vi "mrq_getdi.vi"(3 "错误输入（无错误）":errorcluster, 6 "VISA资源名称":refnum<visa-resource-name>) -> (0 "错误输出":errorcluster, 1 "数字":i32, 2 "VISA资源名称输出":refnum<visa-resource-name>)   [LabVIEW 2017]
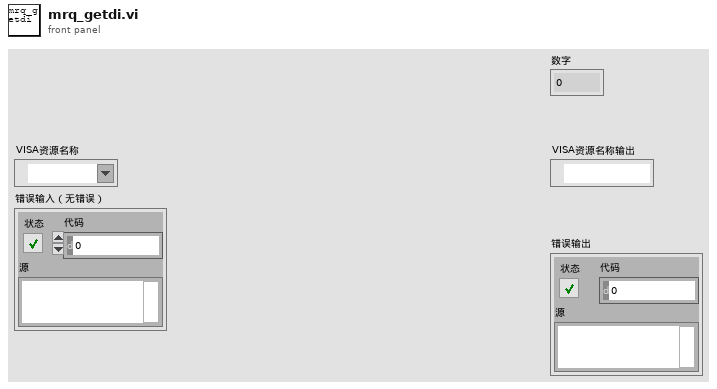
[diagram p1: front panel]
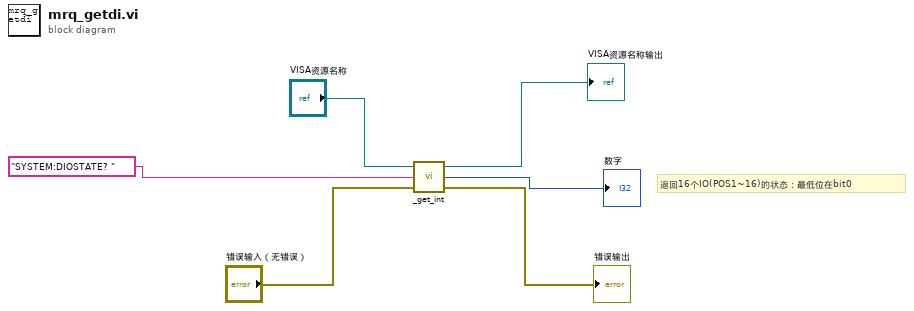
[diagram p0: block diagram]
diagram:
  # "返回16个IO(POS1~16)的状态：最低位在bit0"
  n1 = call "_get_int.vi"("错误输入（无错误）"="错误输入（无错误）", "写入缓冲区"="SYSTEM:DIOSTATE? ", "VISA资源名称"="VISA资源名称") -> ("错误输出"=→"错误输出":errorcluster, "数字"=→"数字":i32, "VISA资源名称输出"=→"VISA资源名称输出":refnum<visa-resource-name>)
